vi "pam model without disturbance.vi"() -> ()   [LabVIEW 2019]
uses:
  <vilib>/Simulation/Implementation/Shared/SIMSCR Execution Mode.ctl
  <vilib>/Simulation/Scripting/Companion Diagram/SimConfigNode/SimParams.ctl
  <vilib>/Simulation/Scripting/Companion Diagram/SimConfigNode/_simSolvers.ctl
  <vilib>/Simulation/Param Hierarchy/Typedefs/SIMPH Param Control Actions.ctl
  <vilib>/Simulation/Implementation/Shared/SIM limit type.ctl
  <vilib>/Simulation/Implementation/Shared/NILVSim_ParamChanged.vi
  <vilib>/Simulation/Implementation/Shared/NILVSIM_BeginStep.vi
  <vilib>/Simulation/ContinuousLinear/Implementation/NILVSim Integrator new.llb/SIM Integrator distributor (scalar).vi
  <vilib>/Simulation/ContinuousLinear/Implementation/NILVSim Integrator new.llb/SIM Integrator collector (scalar).vi
  <vilib>/Simulation/Implementation/Shared/NILVSim_Manager.vi
  <vilib>/Utility/error.llb/Clear Errors.vi
  <vilib>/Simulation/Implementation/Shared/NILVSim_FinalizeModel.vi
  <vilib>/Simulation/Implementation/Shared/SIM Unbundle Sim Info.vi
  <vilib>/Simulation/Implementation/Shared/SIMSH Read Queue.vi
  <vilib>/Simulation/Implementation/Shared/NILVSim_Initialize.vi
  <vilib>/Simulation/Utility/Implementation/NILVSim Get Time and IsAcceptedStep.vi
  <vilib>/Simulation/Implementation/Shared/NILVSim_GetModelError.vi
  <vilib>/Simulation/Implementation/Shared/SIM SimErrorHandler.vi
  <vilib>/Simulation/Implementation/Shared/SIM Bundle Sim Info.vi
  <vilib>/Simulation/Scripting/Companion Diagram/SimConfigNode/SimDog.xnode
  <vilib>/Simulation/Implementation/XNodeFramework/SimXNode/SimX.xnode
  <vilib>/Simulation/ContinuousLinear/Implementation/NILVSim Integrator new.llb/SIM Integrator (scalar).vi
  <vilib>/Simulation/Implementation/Shared/NI_SIM_Implementation.lvlib
panel:
  in  "g":dbl
  in  "m":dbl
  in  "k1":dbl
  in  "k0":dbl
  in  "b1":dbl
  in  "b0":dbl
  in  "f1":dbl
  in  "f0":dbl
  out "output Position":dbl
  in  "Initial Velocity":dbl
  in  "Initial Position":dbl
  in  "Input Pressure":dbl(slide) scale=0.0..10.0
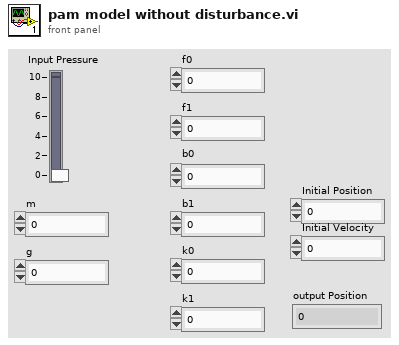
[diagram p1: front panel]
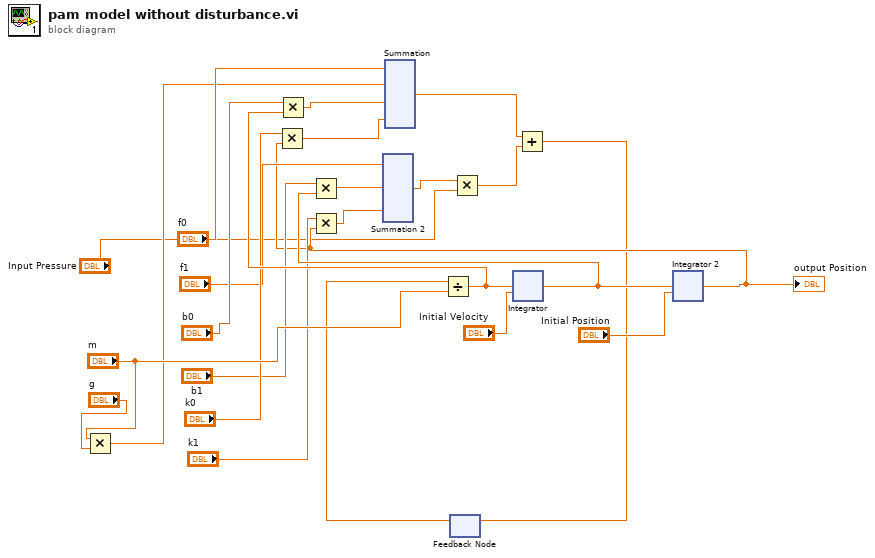
[diagram p0: block diagram]
diagram:
  n1 = Multiply(x="m", y="g") -> (x*y=w19:dbl)
  n2 = feedback #1() -> (w1:dbl)  [unwired: 1 in]
  n3 = Divide(x=w1, y="m") -> (x/y=w15:dbl)
  n4 = Multiply ("Multiply 2")(x="b0", y=w15) -> (x*y=w18:dbl)
  n5 = xnode "Integrator"("input"=w15, "initial condition"="Initial Velocity") -> ("output"=w8:dbl)  [unwired: 8 in, 2 out]
  n6 = Multiply ("Multiply 4")(x="b1", y=w8) -> (x*y=w12:dbl)
  n7 = xnode ("Integrator 2")("input"=w8, "initial condition"="Initial Position") -> ("output"=w6:dbl)  [unwired: 8 in, 2 out]
  "output Position" <- w6
  n8 = Multiply ("Multiply 3")(x="k0", y=w6) -> (x*y=w17:dbl)
  n9 = Multiply ("Multiply 5")(x="k1", y=w6) -> (x*y=w11:dbl)
  n10 = xnode ("Summation 2")("Operand1"="f1", "Operand2"=w12, "Operand3"=w11) -> ("Result"=w10:dbl)
  n11 = xnode ("Summation")("Operand1"="f0", "Operand2"=w19, "Operand3"=w18, "Operand4"=w17) -> ("Result"=w4:dbl)
  n12 = Multiply ("Multiply 6")(x=w10, y="Input Pressure") -> (x*y=w3:dbl)
  n13 = Add(x=w4, y=w3) -> (x+y=w2:dbl)
  n14 = feedback-in #1 ("2")(w2) -> ()
